vi "edit VI constants.vi"(8 "error in":errorcluster, 10 "relative path of VI to edit":path, 11 "custom device path":path=path "C:/Users/nitest/Documents/LabVIEW Data") -> (0 "error out":errorcluster, 3 "custom device path out":path=path "C:/Users/nitest/Documents/LabVIEW Data")   [LabVIEW 2020, in "Template Tool.lvlib"]
uses:
  Template Tool.lvlib
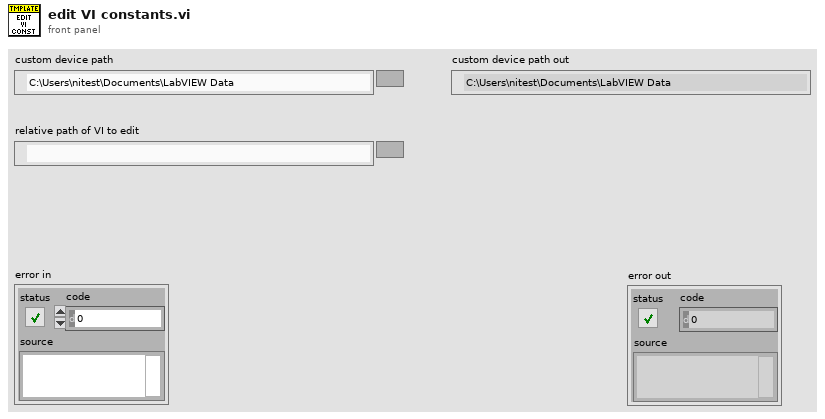
[diagram p1: front panel]
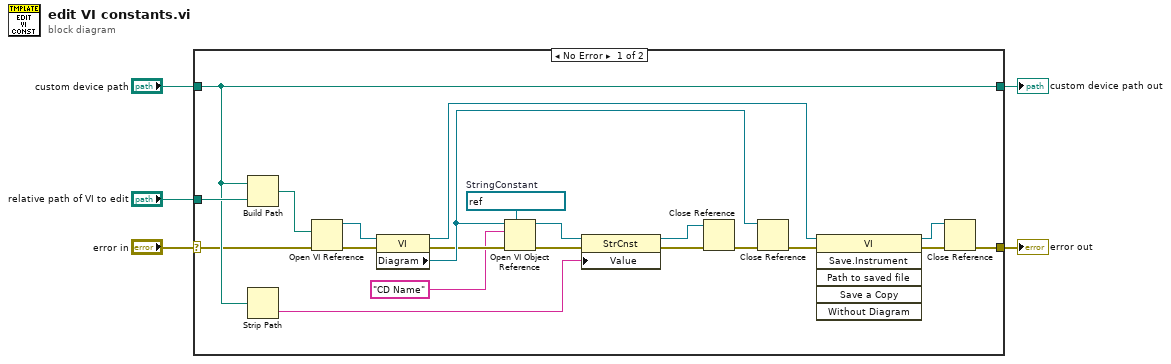
[diagram p0: block diagram]
diagram:
  n1 = case shown="No Error" "error in" {
    selector: "error in" -> [w20 w27]
    tunnel: [w12 w27] -> w5
    tunnel: "custom device path" -> [w21 w28]
    tunnel: "relative path of VI to edit" -> [w22 _]
    tunnel: [w21 w28] -> w2
    frame No Error {
      w9 = refnum<vi> refnum  # StringConstant
      n2 = Build Path(base path=w21, name or relative path=w22) -> (appended path=w24:path)
      n3 = Strip Path(path=w21) -> (name=w19:string)  [unwired: 1 out]
      n4 = Open VI Reference(vi path=w24, error in (no error)=w20) -> (vi reference=w25:refnum<vi>, error out=w26:errorcluster)  [unwired: 4 in]
      n5 = property class="VI"(reference=w25, error in=w26) -> (reference out=w23:refnum<vi>, error out=w11:errorcluster, "Diagram"=w17:refnum<vi>)
      n6 = Open VI Object Reference(7:w9, 8:w11, 10:"CD Name" ("Class Name"), 11:w17) -> (0:w8:errorcluster, 3:w7:refnum<vi>)
      n7 = property class="StrCnst"(reference=w7, error in=w8, "Value"=w19) -> (reference out=w6:refnum<vi>, error out=w16:errorcluster)
      n8 = Close Reference(reference=w6, error in (no error)=w16) -> (error out=w18:errorcluster)
      n9 = Close Reference(reference=w17, error in (no error)=w18) -> (error out=w15:errorcluster)
      n10 = invoke class="VI" method="Save.Instrument"(reference=w23, error in=w15) -> (reference out=w14:refnum<vi>, error out=w13:errorcluster)  [unwired: 4 in, 4 out]
      n11 = Close Reference(reference=w14, error in (no error)=w13) -> (error out=w12:errorcluster)
    }
    frame Error {
    }
  }
  "error out" <- w5
  "custom device path out" <- w2
